vi "Vessel(Port).vi"(10 "Port Number":i32=8500) -> (0 "error out":errorcluster, 1 "TCPConRefJoystick":refnum<k5>, 2 "TCPConRefRecvMsg":refnum<k5>, 3 "Vessel.lvclass":refnum<class "Vessel.lvclass">, 4 "TCPSendArray":refnum<k5>[](array[refnum]))   [LabVIEW 2014, in "Vessel.lvclass"]
uses:
  Vessel.lvclass
  Thrust Allocation/Thrust Allocation().vi
  Thrust Allocation/Thrust Allocation.lvclass
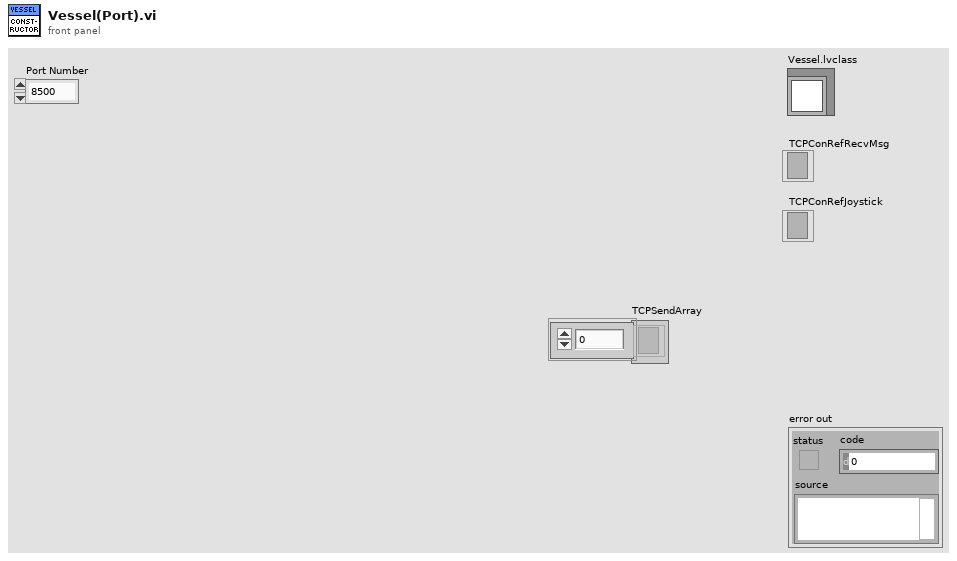
[diagram p1: front panel]
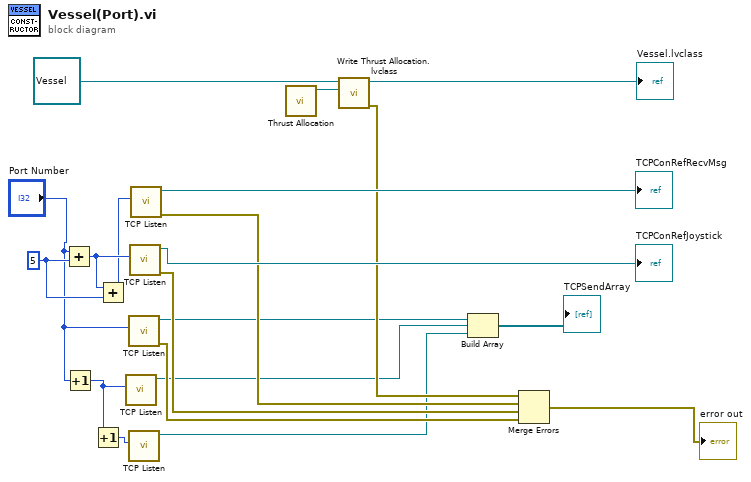
[diagram p0: block diagram]
diagram:
  w19 = 5
  n1 = Add(x="Port Number", y=w19) -> (x+y=w2:i32)
  n2 = Increment(x="Port Number") -> (x+1=w3:i32)
  n3 = Increment(x=w3) -> (x+1=w4:i32)
  n4 = Add(x=w2, y=w19) -> (x+y=w1:i32)
  n5 = call <vilib>:"TCP Listen.vi"("port"=w3) -> ("connection ID"=w7:refnum<k5>)  [unwired: 6 in, 4 out]
  n6 = call <vilib>:"TCP Listen.vi"("port"="Port Number") -> ("error out"=w11:errorcluster, "connection ID"=w9:refnum<k5>)  [unwired: 6 in, 3 out]
  n7 = call <vilib>:"TCP Listen.vi"("port"=w4) -> ("connection ID"=w6:refnum<k5>)  [unwired: 6 in, 4 out]
  n8 = call <vilib>:"TCP Listen.vi"("port"=w2) -> ("error out"=w12:errorcluster, "connection ID"=→"TCPConRefJoystick":refnum<k5>)  [unwired: 6 in, 3 out]
  n9 = call <vilib>:"TCP Listen.vi"("port"=w1) -> ("error out"=w13:errorcluster, "connection ID"=→"TCPConRefRecvMsg":refnum<k5>)  [unwired: 6 in, 3 out]
  n10 = call-poly "Thrust Allocation.vi"() -> ("Thrust Allocation Out"=w18:refnum<class "Thrust Allocation.lvclass">)  [unwired: 11 in]
  n11 = call "Write Thrust Allocation.lvclass.vi"("Thrust Allocation.lvclass"=w18, "Vessel in"=refnum<class "Vessel.lvclass"> refnum ("Vessel.lvclass")) -> ("error out"=w14:errorcluster, "Vessel out"=→"Vessel.lvclass":refnum<class "Vessel.lvclass">)  [unwired: 8 in]
  n12 = Build Array(w9, w7, w6) -> (→"TCPSendArray":refnum<k5>[])
  n13 = Merge Errors(w14, w13, w12, w11) -> (→"error out":errorcluster)
